vi "TeleOp.vi"(10 "Move Arm":dbl, 11 "arm.lvclass":refnum<class "arm.lvclass">) -> (3 "arm.lvclass":refnum<class "arm.lvclass">)   [LabVIEW 2015, in "arm.lvclass"]
uses:
  arm.lvclass
  arm.lvclass/arm.ctl
  Robot Global Data.vi
  <vilib>/addons/control/pid/NI_PID_pid.lvlib
  <vilib>/addons/control/pid/pid.llb/PID Output Rate Limiter (DBL).vi
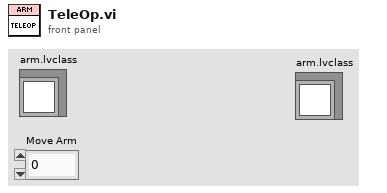
[diagram p1: front panel]
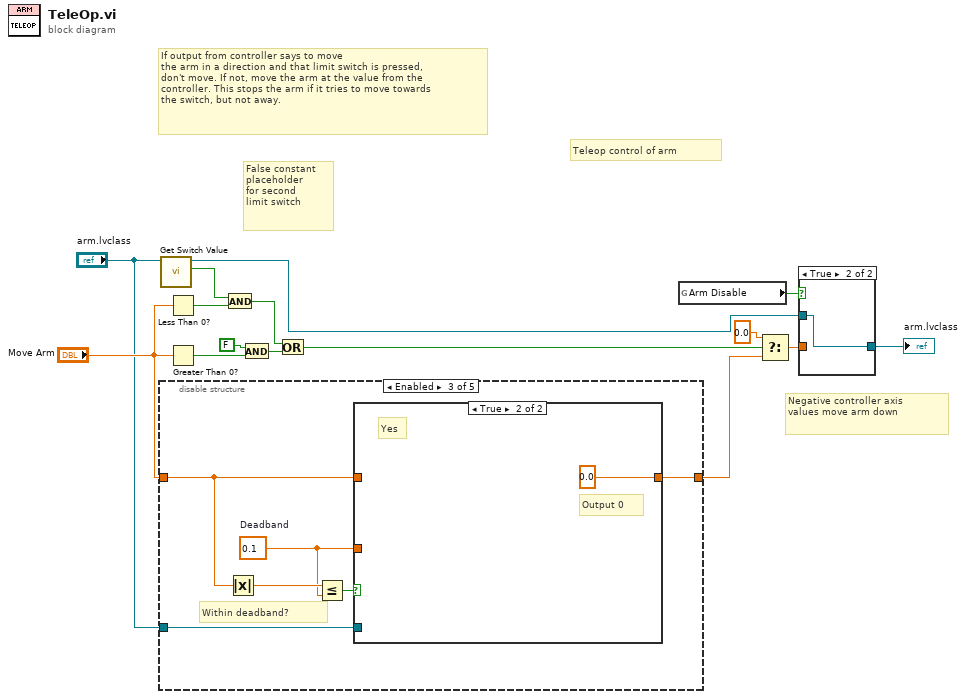
[diagram p0: block diagram]
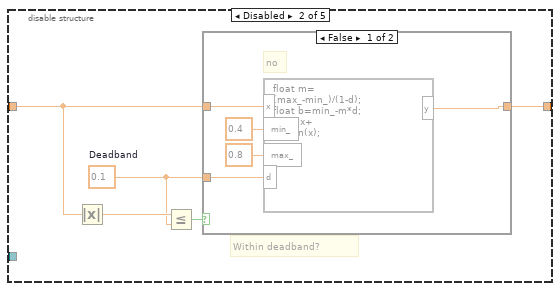
[diagram p3: hidden frame]
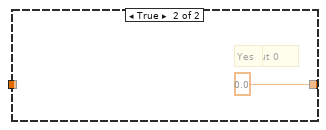
[diagram p4: hidden frame]
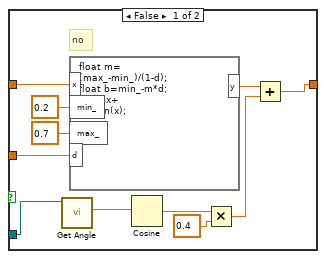
[diagram p5: hidden frame]
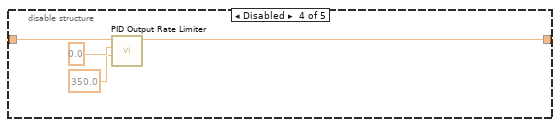
[diagram p6: hidden frame]
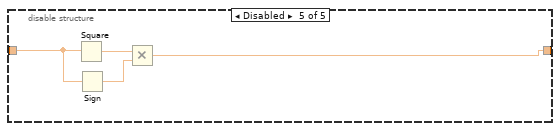
[diagram p7: hidden frame]
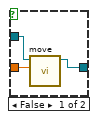
[diagram p8: hidden frame]
diagram:
  # "Teleop control of arm"
  # "If output from controller says to move \nthe arm in a direction and that limit switch is pressed,\ndon't move. If not, move the arm at the value from the\ncontroller. This stops the arm if it tries to move towards\nthe switch, but not away."
  # "False constant \nplaceholder\nfor second \nlimit switch"
  # "Negative controller axis\nvalues move arm down"
  n1 = disable-structure shown="Enabled" {
    disable-tunnel: [w16 w17 w29 w49 w50] -> w8
    disable-tunnel: "Move Arm" -> [w16 w18 w30 w48 w53]
    disable-tunnel: "arm.lvclass" -> [_ _ w28 _ _]
    frame Disabled {
    }
    frame Disabled {
      w19 = 0.1  # Deadband
      # "Within deadband?"
      n2 = Absolute Value(x=w18) -> (abs(x)=w21:dbl)
      n3 = Less Or Equal?(x=w21, y=w19) -> (x <= y?=w20:bool)
      n4 = case shown="False" w20 {
        tunnel: [w26 0.0 ("y")] -> w17
        tunnel: w18 -> [w23 _]
        tunnel: w19 -> [w22 _]
        frame False {
          # "no"
          n5 = formula code="float m= \n(max_-min_)/(1-d);\nfloat b=min_-m*d;\ny=m*x+\nb*sign(x);"("x"=w23, "min_"=0.4 ("input variable"), "max_"=0.8 ("input variable"), "d"=w22) -> ("y"=w26:dbl)
        }
        frame True {
          # "Yes"
          # "Output 0"
        }
      }
    }
    frame Enabled {
      w31 = 0.1  # Deadband
      # "Within deadband?"
      n6 = Absolute Value(x=w30) -> (abs(x)=w33:dbl)
      n7 = Less Or Equal?(x=w33, y=w31) -> (x <= y?=w32:bool)
      n8 = case shown="True" w32 {
        tunnel: [w36 0.0 ("y")] -> w29
        tunnel: w30 -> [w42 _]
        tunnel: w31 -> [w41 _]
        tunnel: w28 -> [w34 _]
        frame False {
          # "no"
          n9 = call "Get Angle.vi"("arm in"=w34) -> ("Angle"=w35:dbl)  [unwired: 9 in, 1 out]
          n10 = formula code="float m= \n(max_-min_)/(1-d);\nfloat b=min_-m*d;\ny=m*x+\nb*sign(x);"("x"=w42, "min_"=0.2 ("input variable"), "max_"=0.7 ("input variable"), "d"=w41) -> ("y"=w38:dbl)
          n11 = Cosine(x=w35) -> (cos(x)=w40:dbl)
          n12 = Multiply(x=w40, y=0.4) -> (x*y=w37:dbl)
          n13 = Add(x=w38, y=w37) -> (x+y=w36:dbl)
        }
        frame True {
          # "Yes"
          # "Output 0"
        }
      }
    }
    frame Disabled {
      n14 = call-poly <vilib>:"PID Output Rate Limiter.vi"("output rate (EGU/min)"=350.0, "initial output"=0.0, "input (controller output)"=w48) -> ("output"=w49:dbl)  [unwired: 5 in, 1 out]
    }
    frame Disabled {
      n15 = Square(x=w53) -> (x^2=w51:dbl)
      n16 = Sign(1:w53) -> (0:w52:dbl)
      n17 = Multiply(x=w51, y=w52) -> (x*y=w50:dbl)
    }
  }
  n18 = call "Get Switch Value.vi"("arm.lvclass"="arm.lvclass") -> ("Switch Pressed"=w5:bool, "arm.lvclass"=w2:refnum<class "arm.lvclass">)  [unwired: 9 in]
  n19 = Less Than 0?(x="Move Arm") -> (x < 0?=w15:bool)
  n20 = Greater Than 0?(x="Move Arm") -> (x > 0?=w14:bool)
  n21 = And(x=w5, y=w15) -> (x .and. y?=w12:bool)
  n22 = And(x=FALSE, y=w14) -> (x .and. y?=w13:bool)
  n23 = Or(x=w12, y=w13) -> (x .or. y?=w11:bool)
  n24 = global read "Robot Global Data.vi" "Arm Disable"() -> (w7:bool)
  n25 = Select(t=0.0, s=w11, f=w8) -> (s? t:f=w10:dbl)
  n26 = case shown="True" w7 {
    tunnel: w10 -> [w56 _]
    tunnel: w2 -> [w55 w57]
    tunnel: [w54 w57] -> w1
    frame False {
      n27 = call "move.vi"("Speed"=w56, "arm.lvclass"=w55) -> ("arm.lvclass"=w54:refnum<class "arm.lvclass">)  [unwired: 9 in]
    }
    frame True {
    }
  }
  "arm.lvclass" <- w1
